vi "Set Largest Decoration Visible (Helper).vi"   [LabVIEW 2015, in "Utility.lvlib"]
uses:
  Utility.lvlib
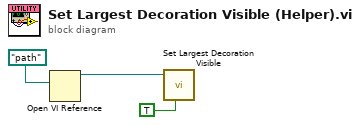
[diagram p0: block diagram]
diagram:
  n1 = Open VI Reference(vi path=path "path") -> (vi reference=w1:refnum<vi>)  [unwired: 5 in, 1 out]
  n2 = call "Set Largest Decoration Visible.vi"("Visible"=TRUE, "VI Ref (calling VI)"=w1) -> ()  [unwired: 8 in, 2 out]
